vi "MoveAfterReference.vi"(8 "error in (no error)":errorcluster, 9 "Position":dbl, 10 "AxisNumber":u8, 11 "CS++Motor in":refnum<class "CS++Motor.lvclass">) -> (0 "error out":errorcluster, 3 "CS++Motor out":refnum<class "CS++Motor.lvclass">)   [LabVIEW 2015, in "CS++Motor.lvlib" / "CS++Motor.lvclass"]
doc: "Starts a movement to the reference switch of this axis. Once the motor reaches the reference switch it should slowly move down from the switch, resets the internal step counter and moves to the desired absolute position.\n\nThis function is a combination of <b>Move.vi</b> and <b>ReferenceMove.vi</b>."
uses:
  CS++Motor.lvclass
  CS++Motor.lvclass/CS++Motor.ctl
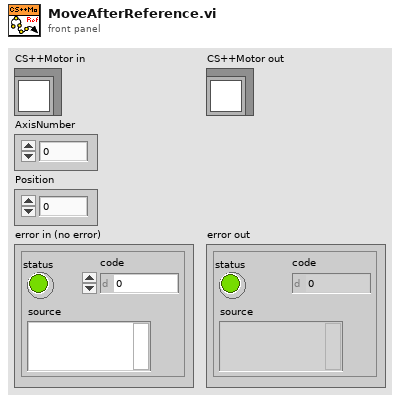
[diagram p1: front panel]
types:
  T1 = cluster{"LogicalName":string, "PhysicalName":string, "unit":string, "Scaling":dbl, "SetPosition":dbl, "RawSetPosition":dbl, "StartVelocity":dbl, "StopVelocity":dbl, "Acceleration":dbl, "RangeMin":dbl, "RangeMax":dbl, "LogicalPos-Array":cluster{"LogicalPosition":string, "SetPosition":dbl}[]}[]
  T2 = cluster{"LogicalName":string, "PhysicalName":string, "unit":string, "Scaling":dbl, "SetPosition":dbl, "RawSetPosition":dbl, "StartVelocity":dbl, "StopVelocity":dbl, "Acceleration":dbl, "RangeMin":dbl, "RangeMax":dbl, "LogicalPos-Array":cluster{"LogicalPosition":string, "SetPosition":dbl}[]}
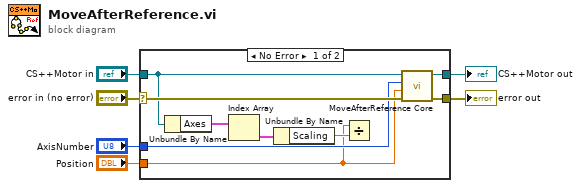
[diagram p0: block diagram]
diagram:
  n1 = case shown="No Error" "error in (no error)" {
    selector: "error in (no error)" -> [w14 w17]
    tunnel: [w13 w17] -> w5
    tunnel: [w15 w16] -> w3
    tunnel: "CS++Motor in" -> [w8 w16]
    tunnel: "AxisNumber" -> [w12 _]
    tunnel: "Position" -> [w7 _]
    frame No Error {
      n2 = Unbundle By Name(w8) -> ("Axes"=w11:T1)
      n3 = Index Array(array=w11) -> (element=w10:T2)  [unwired: 1 in]
      n4 = Unbundle By Name(w10) -> ("Scaling"=w9:dbl)
      n5 = Divide(x=w7, y=w9) -> ()  [unwired: 1 out]
      n6 = call-dynamic "MoveAfterReference Core.vi"("error in (no error)"=w14, "Raw-Position"=w7, "AxisNumber"=w12, "CS++Motor in"=w8) -> ("error out"=w13:errorcluster, "CS++Motor out"=w15:refnum<class "CS++Motor.lvclass">)  [unwired: 6 in]
    }
    frame Error {
    }
  }
  "error out" <- w5
  "CS++Motor out" <- w3
